vi "Read.vi"(8 "error in":errorcluster, 10 "task/channels in":refnum<k21>, 11 "4-20mA Settings Input":T1) -> (0 "error out":errorcluster, 1 "Connection Error":bool, 2 "Read":dbl, 3 "4-20mA Settings Output":T1)   [LabVIEW 2018, in "Pressure Transmitter Library.lvlib"]
uses:
  Pressure Transmitter Library.lvlib
  Pressure Transmitter Device Settings.ctl
  <vilib>/DAQmx/read.llb/DAQmx Read (Analog DBL 1Chan 1Samp).vi
  <vilib>/DAQmx/miscellaneous.llb/DAQmx Fill In Error Info.vi
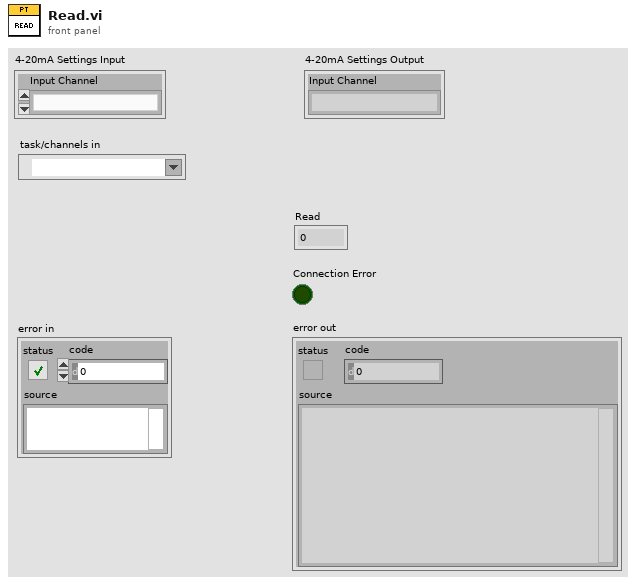
[diagram p1: front panel]
types:
  T1 = typedef "Pressure Transmitter Library.lvlib/Pressure Transmitter Device Settings.ctl" = cluster{"Input Channel ":u16}
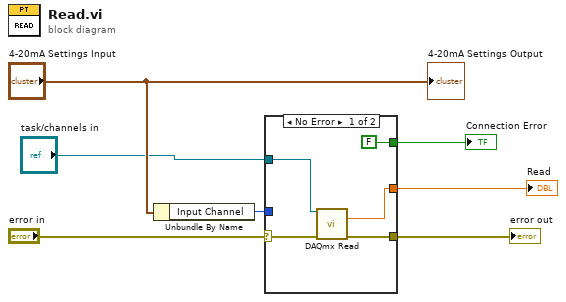
[diagram p0: block diagram]
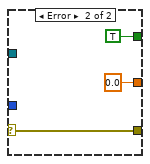
[diagram p2: hidden frame]
diagram:
  n1 = Unbundle By Name("4-20mA Settings Input") -> ("Input Channel"=w6:u16)
  n2 = case shown="No Error" "error in" {
    selector: "error in" -> [w11 w14]
    tunnel: w6 -> [_ _]
    tunnel: [w12 w14] -> w5
    tunnel: [FALSE ("Pump On?") TRUE ("Pump On?")] -> w2
    tunnel: [w10 0.0 ("data")] -> w3
    tunnel: "task/channels in" -> [w8 _]
    frame No Error {
      n3 = call-poly <vilib>:"DAQmx Read.vi"("task/channels in"=w8, "error in"=w11) -> ("data"=w10:dbl, "error out"=w12:errorcluster)  [unwired: 11 in, 1 out]
    }
    frame Error {
    }
  }
  "error out" <- w5
  "Connection Error" <- w2
  "Read" <- w3
  "4-20mA Settings Output" <- "4-20mA Settings Input"
